vi "programa 10.vi"() -> ()   [LabVIEW 2011]
uses:
  Control del programa 10.ctl
panel:
  out "Array":dbl[][](array[numeric])
  # "Se debera de ingresar datos en todas las lineas dejando la ultima columna\nreservado para la suma de cada una de las lineas y guardando la suma en la ultima columna."
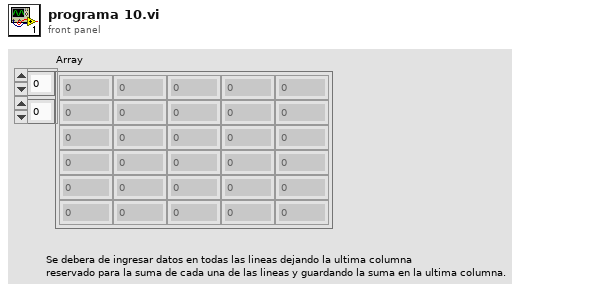
[diagram p1: front panel]
types:
  T1 = typedef "Control del programa 10.ctl" = enum16{"Inicializar", "Rellenar", "Sumar lineas", "Finalizar"}
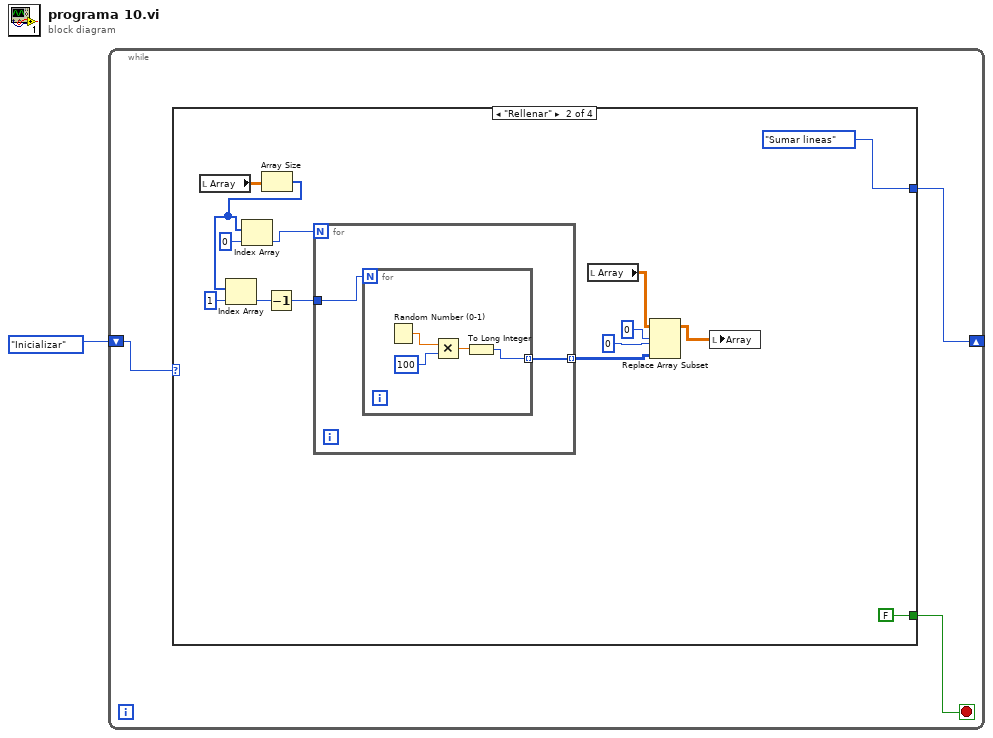
[diagram p0: block diagram]
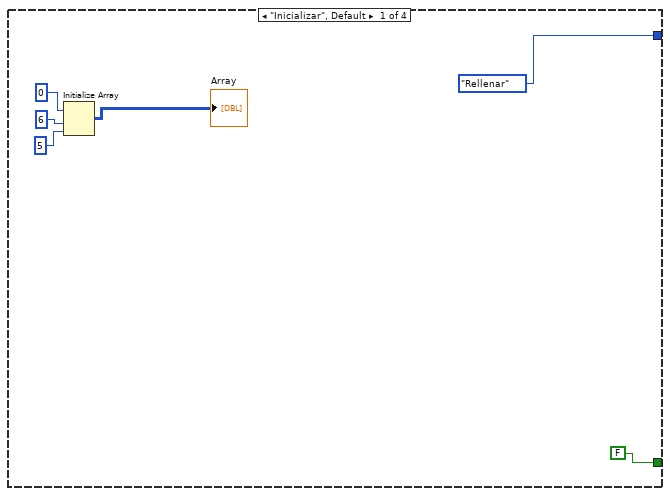
[diagram p2: hidden frame]
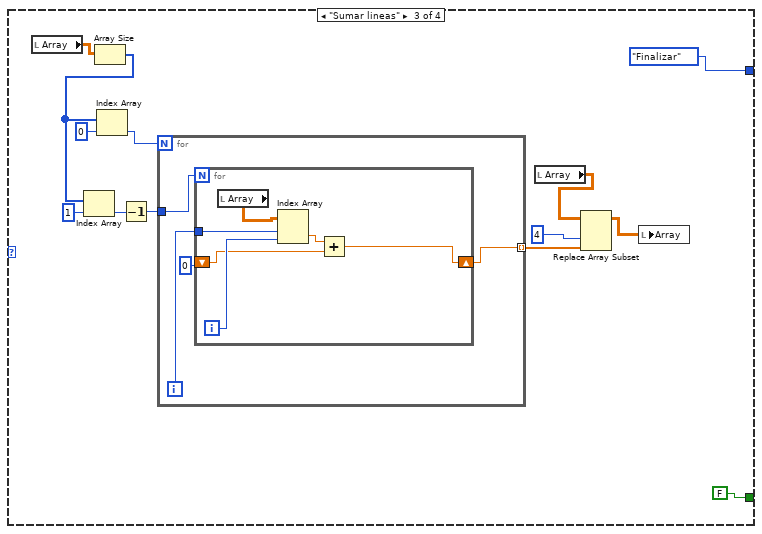
[diagram p3: hidden frame]
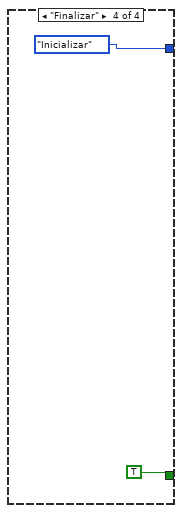
[diagram p4: hidden frame]
diagram:
  n1 = while {
    shift-right: [w3] -> _
    shift-left: Control_del_programa_10."Inicializar" -> [w4]
    stop <- w2 stop-if-true
    n2 = case shown="\"Rellenar\"" w4 {
      tunnel: [Control_del_programa_10."Rellenar" Control_del_programa_10."Sumar lineas" Control_del_programa_10."Finalizar" Control_del_programa_10."Inicializar"] -> w3
      tunnel: [FALSE FALSE FALSE TRUE] -> w2
      frame "Inicializar", Default {
        n3 = Initialize Array "Initialize Array"(0, 6, 5) -> (→"Array":i32[][])
      }
      frame "Rellenar" {
        n4 = local read "Array"() -> (w22:dbl[][])
        n5 = Array Size(array=w22) -> (size(s)=w19:i32[])
        n6 = Index Array "Index Array"(array=w19, index=1) -> (element=w17:i32)
        n7 = Index Array "Index Array"(array=w19, index=0) -> (element=w20:i32)
        n8 = Decrement(x=w17) -> (x-1=w16:i32)
        n9 = for {
          N: w20 -> [_]
          tunnel: w16 -> [w26]
          tunnel: [w25] -> w12 mode=indexing
          n10 = for {
            N: w26 -> [_]
            tunnel: [w27] -> w25 mode=indexing
            n11 = Random Number (0-1)() -> (number: 0 to 1=w29:dbl)
            n12 = Multiply(x=w29, y=100) -> (x*y=w28:dbl)
            n13 = To Long Integer(number=w28) -> (32bit integer=w27:i32)
          }
        }
        n14 = local read "Array"() -> (w15:dbl[][])
        n15 = Replace Array Subset "Replace Array Subset"(array=w15, new element=w12, index (row)=0, index (col)=0) -> (w11:dbl[][])
        n16 = local write "Array"(w11) -> ()
      }
      frame "Sumar lineas" {
        n17 = local read "Array"() -> (w42:dbl[][])
        n18 = Array Size(array=w42) -> (size(s)=w40:i32[])
        n19 = Index Array "Index Array"(array=w40, index=1) -> (element=w38:i32)
        n20 = Index Array "Index Array"(array=w40, index=0) -> (element=w36:i32)
        n21 = Decrement(x=w38) -> (x-1=w37:i32)
        n22 = for {
          N: w36 -> [_]
          tunnel: w37 -> [w47]
          tunnel: [w44] -> w33 mode=indexing
          i -> [w46]
          n23 = for {
            N: w47 -> [_]
            tunnel: w46 -> [w51]
            shift-right: [w48] -> w44
            shift-left: 0 -> [w49]
            i -> [w52]
            n24 = local read "Array"() -> (w53:dbl[][])
            n25 = Index Array "Index Array"(array=w53, index (row)=w51, index (col)=w52) -> (element=w50:dbl)
            n26 = Add(x=w50, y=w49) -> (x+y=w48:dbl)
          }
        }
        n27 = local read "Array"() -> (w35:dbl[][])
        n28 = Replace Array Subset "Replace Array Subset"(array=w35, new element=w33, index (col)=4 ("disabled index (col)")) -> (w34:dbl[][])  [unwired: 1 in]
        n29 = local write "Array"(w34) -> ()
      }
      frame "Finalizar" {
      }
    }
  }
